vi "4_2.vi"() -> ()   [LabVIEW 2023]
panel:
  out "Waveform Graph":dynamicdata(graph)
  in  "Knob":dbl(knob) scale=0.0..100.0
  in  "stop (F)":bool
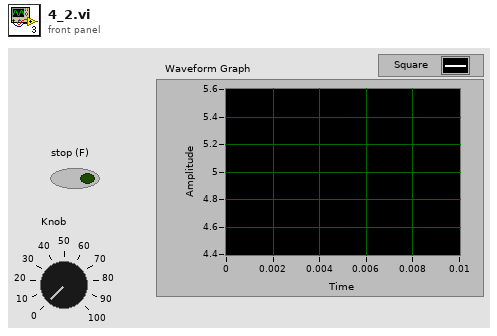
[diagram p1: front panel]
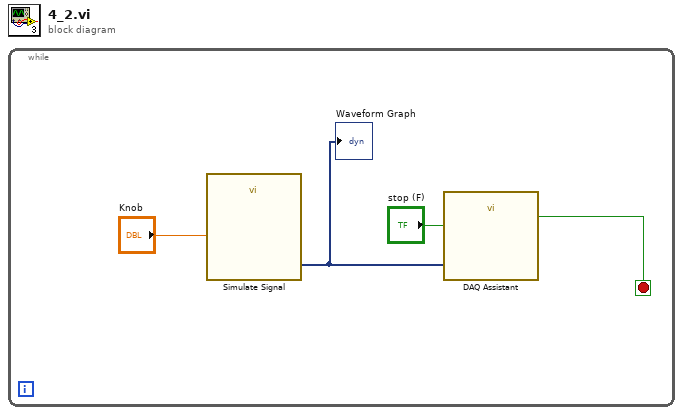
[diagram p0: block diagram]
diagram:
  n1 = while {
    stop <- w3 stop-if-true
    n2 = call "Simulate Signal"("Duty Cycle (%)"="Knob") -> ("Square"=w1:dynamicdata)  [unwired: 13 in, 1 out]
    "Waveform Graph" <- w1
    n3 = call "DAQ Assistant"("data"=w1, "stop (F)"="stop (F)") -> ("stopped"=w3:bool)  [unwired: 15 in, 2 out]
  }
